vi "recording.vi"() -> ()   [LabVIEW 2012]
doc: "This VI will initialize the FPGA VI and read a user-defined number of samples from a DMA FIFO. When the data acquisition is complete this VI will read status information from the FPGA VI.\n\nFollow these instructions to run the VI.\n\n1. Select your RIO device from the dropdown.\n2. Set the sample period, number of samples to acquire per channel, and DMA block read size. \n\nNote: the block read size should be set to balance load on the host processor and the update rate of the user interface. A small block read size will update the user interface more often but will result in a higher load on the host processor."
uses:
  <vilib>/userdefined/High Color/nirio_resource_hc.ctl
  <vilib>/FPGAPlugInAG/sbRIO-9612/niLvFpga_Open_sbRIO-9612.vi
  <vilib>/rvi/interface/common/dynamic/niFpgaDynamicAddResources.vi
  <vilib>/Utility/error.llb/Error Cluster From Error Code.vi
  <vilib>/FPGAPlugInAG/Dynamic/niLvFpga_Run_Dynamic.vi
  <vilib>/rvi/errors/niLvFpgaAdjustHostInterfaceError.vi
  <vilib>/RVI Host/nirviSupport.llb/nirviErrorClusterFromErrorCode.vi
  <vilib>/FPGAPlugInAG/Dynamic/niLvFpga_Close_Dynamic.vi
  <vilib>/rvi/interface/nirviOpenFPGA/nirviOpenFPGA.xnode
  FPGA Bitfiles/bbauvFPGA_FPGATarget2_NI9223User-Contr_AXBjtBmtN8Y.lvbitx
  NI 9223 User-Controlled IO Sampling (FPGA).vi
  <vilib>/rvi/interface/nirviMethod/nirviMethod.xnode
  <vilib>/rvi/interface/nirviReadWriteControl/nirviReadWriteControl.xnode
  <vilib>/rvi/interface/nirviCloseFPGA/nirviCloseFPGA.xnode
  <vilib>/rvi/errors/niLvFpgaMergeErrorWithErrorCode.vi
  <vilib>/rvi/interface/Simulation/niFpgaSimulationCallBeginRW.vi
  <vilib>/FPGAPlugInAG/Dynamic/niLvFpga_ReadFifo_Dynamic.vi
  <vilib>/rvi/interface/nirviMethod/StockFPGA_InlinedMethodWaitForSingleIRQ.vi
  <vilib>/FPGAPlugInAG/Dynamic/niLvFpga_WaitOnIrq_Dynamic.vi
  <vilib>/FPGAPlugInAG/Dynamic/niLvFpga_AcknowledgeIrq_Dynamic.vi
  NiFpgaLv.dll
  <vilib>/FPGAPlugInAG/Dynamic/niLvFpga_ConfigureFifo_Dynamic.vi
  <vilib>/FPGAPlugInAG/Dynamic/niLvFpga_StartFifo_Dynamic.vi
panel:
  in  "Filename":path=path "D/Recorded/US Test/Record 1/test 1.tdms"
  in  "Record?":bool
  out "Waveform Graph":dynamicdata(graph)
  out "Ch0 Signal":sgl[](graph)
  out "#Elements Acquired":u32(graph)
  in  "Sampling Duration (us)":u32=2005000
  in  "RIO Device":T1="rio://192.168.0.150/RIO0"
  out "Timed Out":bool
  out "Sample Gated":bool
  out "Overwrite":bool
  in  "Acquisition Stop":bool
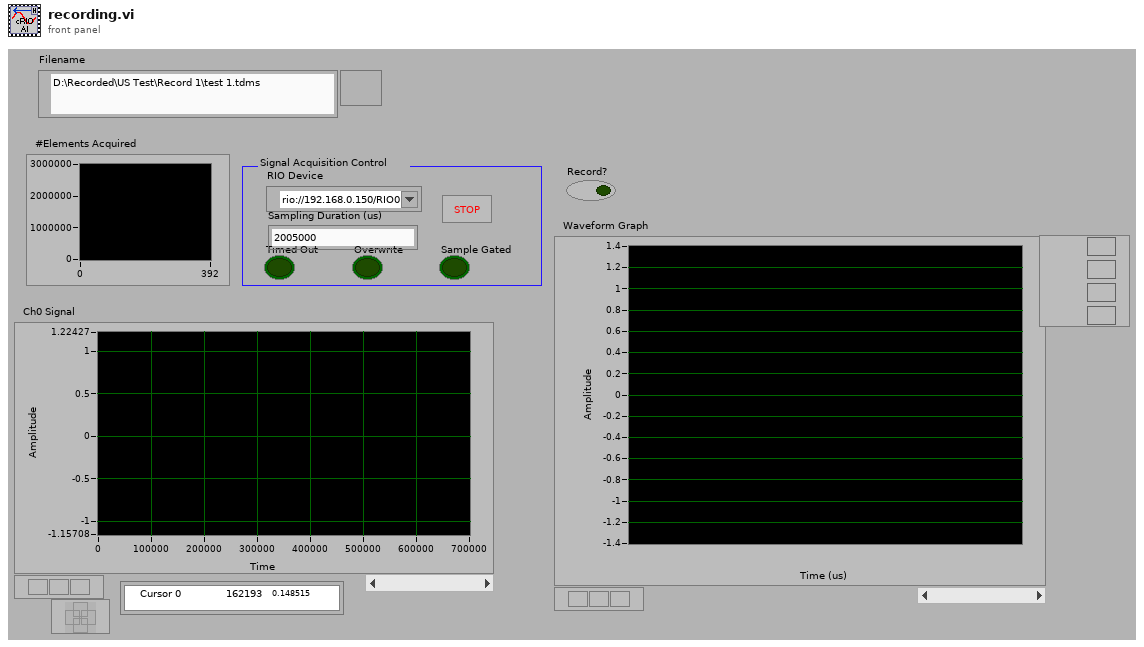
[diagram p1: front panel]
types:
  T1 = typedef "nirio_resource_hc.ctl" = tag
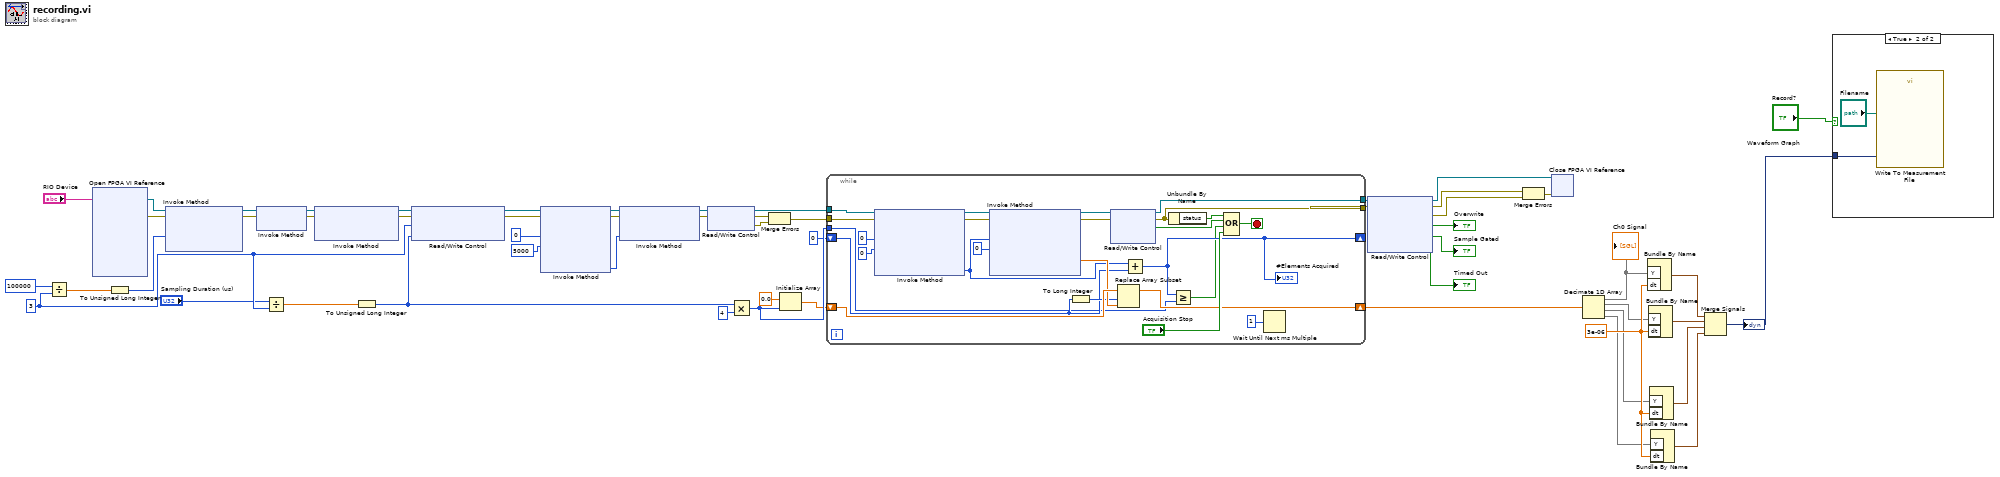
[diagram p0: block diagram]
diagram:
  w9 = 3e-06
  w16 = u32 3
  n1 = Divide(x=u32 100000, y=w16) -> (x/y=w49:dbl)
  n2 = xnode "Open FPGA VI Reference"("resource name"="RIO Device") -> ("FPGA VI Reference Out"=w52:refnum<k20>, "error out"=w51:errorcluster)  [unwired: 1 in]
  n3 = To Unsigned Long Integer(number=w49) -> (unsigned 32bit integer=w50:u32)
  n4 = xnode "Invoke Method"("FPGA VI Reference In"=w52, "error in"=w51, "Requested Depth"=w50) -> ("FPGA VI Reference Out"=w54:refnum<k20>, "error out"=w53:errorcluster)  [unwired: 1 out]
  n5 = xnode "Invoke Method"("FPGA VI Reference In"=w54, "error in"=w53) -> ("FPGA VI Reference Out"=w43:refnum<k20>, "error out"=w42:errorcluster)
  n6 = Divide(x="Sampling Duration (us)", y=w16) -> (x/y=w14:dbl)
  n7 = xnode "Invoke Method"("FPGA VI Reference In"=w43, "error in"=w42) -> ("FPGA VI Reference Out"=w19:refnum<k20>, "error out"=w18:errorcluster)  [unwired: 1 in]
  n8 = To Unsigned Long Integer(number=w14) -> (unsigned 32bit integer=w13:u32)
  n9 = xnode "Read/Write Control"("FPGA VI Reference In"=w19, "error in"=w18, "Sample Period (uSec)"=w16, "Number of Samples"=w13) -> ("FPGA VI Reference Out"=w33:refnum<k20>, "error out"=w32:errorcluster)
  n10 = xnode "Invoke Method"("FPGA VI Reference In"=w33, "error in"=w32, "IRQ Number(s)"=0, "Timeout (ms)"=5000) -> ("FPGA VI Reference Out"=w30:refnum<k20>, "error out"=w31:errorcluster, "IRQ(s) Asserted"=w27:i32)  [unwired: 1 out]
  n11 = xnode "Invoke Method"("FPGA VI Reference In"=w30, "error in"=w31, "IRQ Number(s)"=w27) -> ("FPGA VI Reference Out"=w29:refnum<k20>, "error out"=w28:errorcluster)
  n12 = xnode "Read/Write Control"("FPGA VI Reference In"=w29, "error in"=w28) -> ("FPGA VI Reference Out"=w21:refnum<k20>, "error out"=w35:errorcluster, "Error Out"=w34:errorcluster)
  n13 = Multiply(x=w13, y=u32 4) -> (x*y=w46:u32)
  n14 = Merge Errors(w35, w34) -> (w20:errorcluster)
  n15 = Initialize Array(sgl 0.0, w46) -> (w22:sgl[])
  n16 = while {
    tunnel: w21 -> [w67]
    tunnel: w20 -> [w66]
    tunnel: [w75] -> w41
    tunnel: [w74] -> w40
    shift-right: [w57] -> _
    shift-left: u32 0 -> [w68]
    tunnel: w46 -> [w60]
    shift-right: [w70] -> w1
    shift-left: w22 -> [w76]
    stop <- w77 stop-if-true
    n17 = xnode "Invoke Method"("FPGA VI Reference In"=w67, "error in"=w66, "Number of Elements"=u32 0, "Timeout (ms)"=0) -> ("FPGA VI Reference Out"=w65:refnum<k20>, "error out"=w64:errorcluster, "Elements Remaining"=w58:u32)  [unwired: 1 out]
    n18 = xnode "Invoke Method"("FPGA VI Reference In"=w65, "error in"=w64, "Number of Elements"=w58, "Timeout (ms)"=0) -> ("FPGA VI Reference Out"=w80:refnum<k20>, "error out"=w79:errorcluster, "Data"=w71:sgl[])  [unwired: 1 out]
    n19 = To Long Integer(number=w68) -> (32bit integer=w69:i32)
    n20 = xnode "Read/Write Control"("FPGA VI Reference In"=w80, "error in"=w79) -> ("FPGA VI Reference Out"=w75:refnum<k20>, "error out"=w74:errorcluster, "Error"=w59:bool)  [unwired: 1 out]
    n21 = Replace Array Subset(array=w76, new element=w71, index=w69) -> (w70:sgl[])
    n22 = Add(x=w58, y=w68) -> (x+y=w57:u32)
    "#Elements Acquired" <- w57
    n23 = Unbundle By Name(w74) -> ("status"=w61:bool)
    n24 = Greater Or Equal?(x=w57, y=w60) -> (x >= y?=w56:bool)
    n25 = Compound Arithmetic op=OR(w61, w59, w56, "Acquisition Stop") -> (w77:bool)
    n26 = Wait Until Next ms Multiple(millisecond multiple=u32 1) -> ()  [unwired: 1 out]
  }
  n27 = xnode "Read/Write Control"("FPGA VI Reference In"=w41, "error in"=w40) -> ("FPGA VI Reference Out"=w45:refnum<k20>, "error out"=w36:errorcluster, "Error Out"=w37:errorcluster, "Overwrite"=→"Overwrite":bool, "Sample Gated"=→"Sample Gated":bool, "Timed Out"=→"Timed Out":bool)
  n28 = Merge Errors(w36, w37) -> (w44:errorcluster)
  n29 = xnode "Close FPGA VI Reference"("FPGA VI Reference In"=w45, "error in"=w44) -> ()  [unwired: 1 out]
  n30 = Decimate 1D Array(w1) -> (w2:sgl[], w7:sgl[], w6:sgl[], w5:sgl[])
  "Ch0 Signal" <- w2
  n31 = Bundle By Name("Y"=w2, "dt"=w9) -> (w12:waveform(sgl))  [unwired: 1 in]
  n32 = Bundle By Name("Y"=w7, "dt"=w9) -> (w11:waveform(sgl))  [unwired: 1 in]
  n33 = Bundle By Name("Y"=w6, "dt"=w9) -> (w10:waveform(sgl))  [unwired: 1 in]
  n34 = Bundle By Name("Y"=w5, "dt"=w9) -> (w8:waveform(sgl))  [unwired: 1 in]
  n35 = Merge Signals(w12, w11, w10, w8) -> (w4:dynamicdata)
  "Waveform Graph" <- w4
  n36 = case shown="True" "Record?" {
    tunnel: w4 -> [_ w82]
    frame False {
    }
    frame True {
      n37 = call "Write To Measurement File"("Signals"=w82, "Filename"="Filename") -> ()  [unwired: 15 in, 3 out]
    }
  }
